vi "Get Last File Number.vi"(11 "file path out":path) -> (3 "Number":i32 format="%04d")   [LabVIEW 2024]
panel:
  out "File name without extension":string
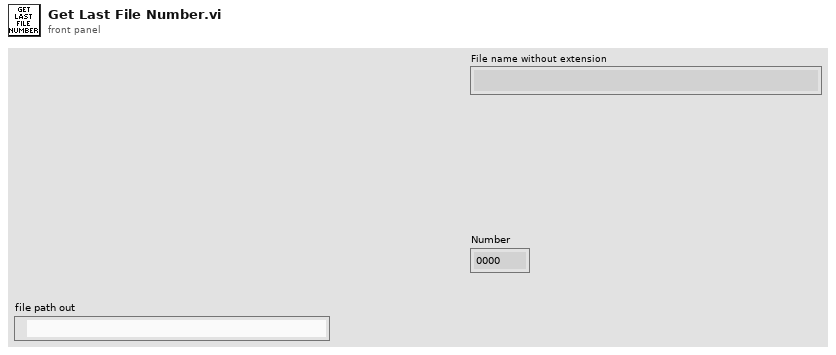
[diagram p1: front panel]
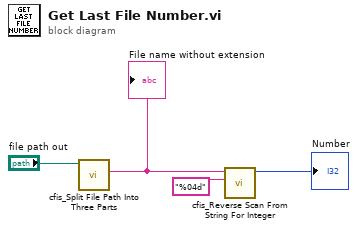
[diagram p0: block diagram]
diagram:
  n1 = call <vilib>:"cfis_Split File Path Into Three Parts.vi"("file path"="file path out") -> ("File name without extension"=w3:string)  [unwired: 8 in, 2 out]
  "File name without extension" <- w3
  n2 = call <vilib>:"cfis_Reverse Scan From String For Integer.vi"("format string"="%04d", "input string"=w3) -> ("Extracted integer"=→"Number":i32)  [unwired: 9 in]
